vi "Send Arm Acquisition Engine.vi"(8 "error in":errorcluster, 11 "FPGA VI Reference In":refnum<k20>) -> (0 "error out":errorcluster, 3 "FPGA VI Reference Out":refnum<k20>)   [LabVIEW 2012]
uses:
  <vilib>/Utility/error.llb/Error Cluster From Error Code.vi
  <vilib>/rvi/errors/niLvFpgaAdjustHostInterfaceError.vi
  <vilib>/rvi/interface/nirviReadWriteControl/nirviReadWriteControl.xnode
  NiFpgaLv.dll
  <vilib>/rvi/interface/Simulation/niFpgaSimulationCallBeginRW.vi
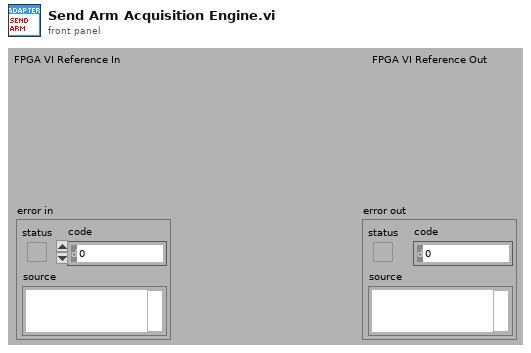
[diagram p1: front panel]
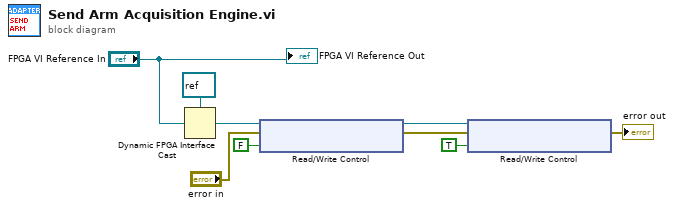
[diagram p0: block diagram]
diagram:
  n1 = Dynamic FPGA Interface Cast(Session In=refnum<k20> refnum ("Type"), Type="FPGA VI Reference In") -> (Session Out=w2:refnum<k20>)
  n2 = xnode "Read/Write Control"("FPGA VI Reference In"=w2, "error in"="error in", "Arm Acquisition Engine"=FALSE ("Reset?")) -> ("FPGA VI Reference Out"=w6:refnum<k20>, "error out"=w5:errorcluster)
  n3 = xnode "Read/Write Control"("FPGA VI Reference In"=w6, "error in"=w5, "Arm Acquisition Engine"=TRUE ("Reset?")) -> ("error out"=→"error out":errorcluster)  [unwired: 1 out]
  "FPGA VI Reference Out" <- "FPGA VI Reference In"
